vi "Wrapper For Assert True.vi"(8 "error in (no error)":errorcluster) -> (0 "error out":errorcluster)   [LabVIEW 2013]
uses:
  classes/Assert/Assert.lvclass
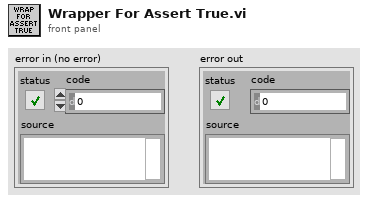
[diagram p1: front panel]
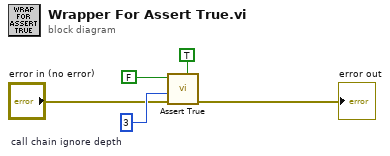
[diagram p0: block diagram]
diagram:
  w3 = 3  # call chain ignore depth
  n1 = call "Assert True.vi"("Assert Only? (F)"=TRUE, "error in (no error)"="error in (no error)", "call chain ignore depth (2)"=w3, "True?"=FALSE) -> ("error out"=→"error out":errorcluster)  [unwired: 7 in]
